vi "DMMP_GetInstrumentHandle.vi"(3 "Input DMMP":refnum<class "DMMP.lvclass">) -> (0 "DMM Serial Port":refnum<visa-resource-name>, 1 "Output DMMP":refnum<class "DMMP.lvclass">)   [LabVIEW 2014, in "DMMP.lvclass"]
uses:
  DMMP.lvclass
  DMMP.lvclass/DMMP.ctl
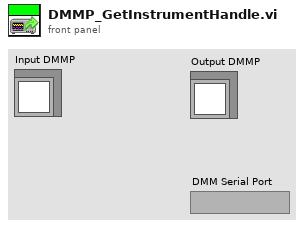
[diagram p1: front panel]
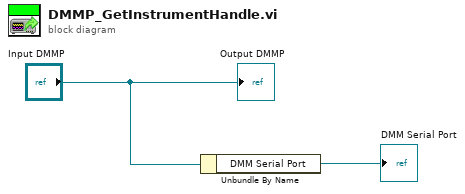
[diagram p0: block diagram]
diagram:
  n1 = Unbundle By Name("Input DMMP") -> ("DMM Serial Port"=→"DMM Serial Port":refnum<visa-resource-name>)
  "Output DMMP" <- "Input DMMP"
